vi "Set Exclusions.vi"(4 "Exclude dependent shared libraries":bool, 6 "Exclude dependent packed libraries":bool, 8 "error in (no error)":errorcluster, 9 "Disconnect inline subVIs":bool, 10 "Exclusions":T1={"Disconnect type definitions"=FALSE, "Remove unused polymorphic VI instances"=TRUE, "Remove unused members of project libraries"=TRUE, "Modify project library file after removing unused members"=TRUE}, 11 "Build in":refnum<class "NI_AB_API_Build.lvclass">) -> (0 "error out":errorcluster, 3 "Build out":refnum<class "NI_AB_API_Build.lvclass">)   [LabVIEW 2020, in "NI_AB_API_Build.lvclass"]
uses:
  <vilib>/AppBuilder/AB_API/Build/NI_AB_API_Build.lvclass
  <vilib>/AppBuilder/AB_API/common/AB_API Primary Exclusions.ctl
  <vilib>/AppBuilder/AB_API/Build/NI_AB_API_Build.lvclass/NI_AB_API_Build.ctl
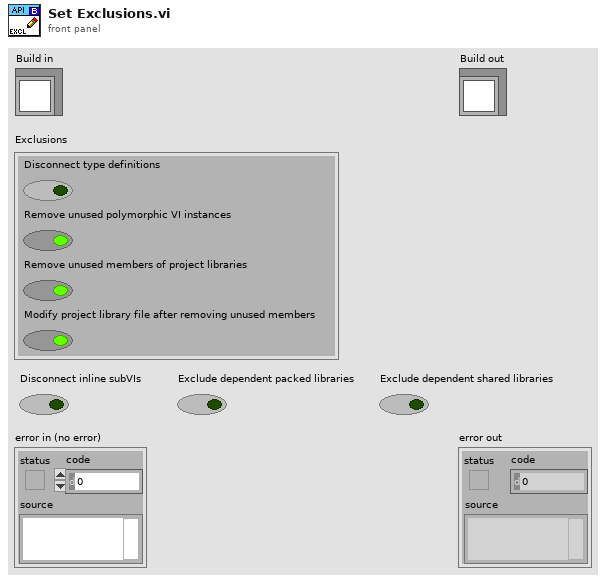
[diagram p1: front panel]
types:
  T1 = typedef "AB_API Primary Exclusions.ctl" = cluster{"Disconnect type definitions":bool, "Remove unused polymorphic VI instances":bool, "Remove unused members of project libraries":bool, "Modify project library file after removing unused members":bool}
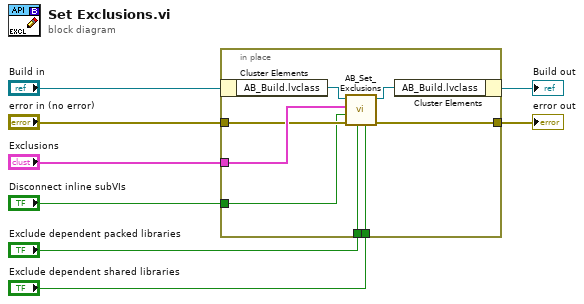
[diagram p0: block diagram]
diagram:
  n1 = in-place {
    in-place-border: "Exclusions" -> [w16]
    in-place-border: "error in (no error)" -> [w15]
    in-place-border: [w14] -> w7
    in-place-border: "Disconnect inline subVIs" -> [w11]
    in-place-border: "Exclude dependent packed libraries" -> [w10]
    in-place-border: "Exclude dependent shared libraries" -> [w9]
    n2 = in-place-cluster #1("Build in") -> ("AB_Build.lvclass"=w13:refnum<class "AB_Build.lvclass">)
    n3 = call <vilib>:"AB_Set_Exclusions.vi"("Exclude dependent shared libraries"=w9, "Exclude dependent packed libraries"=w10, "error in (no error)"=w15, "Disconnect inline subVIs"=w11, "Exclusions"=w16, "Build in"=w13) -> ("error out"=w14:errorcluster, "Build out"=w12:refnum<class "AB_Build.lvclass">)  [unwired: 4 out]
    n4 = in-place-cluster #1("AB_Build.lvclass"=w12) -> (→"Build out":refnum<class "NI_AB_API_Build.lvclass">)
  }
  "error out" <- w7
